vi "CmdExe.Run SystemExec and Wait, with Timeout.vi"() -> ()   [LabVIEW 2018]
uses:
  CmdConsole/CmdConsole.lvclass
  <vilib>/KATE/Time/Time Utils.lvlib
panel:
  out "Duration":dbl
  out "Std Out":string
  out "RtnCode":i32
  out "Std Error":string
  in  "Timeout(s)":dbl=1.0
  out "WaitForExit":bool
  out "HasExited":bool
  in  "Args":string
  out "error out":errorcluster
  in  "error in (no error)":errorcluster
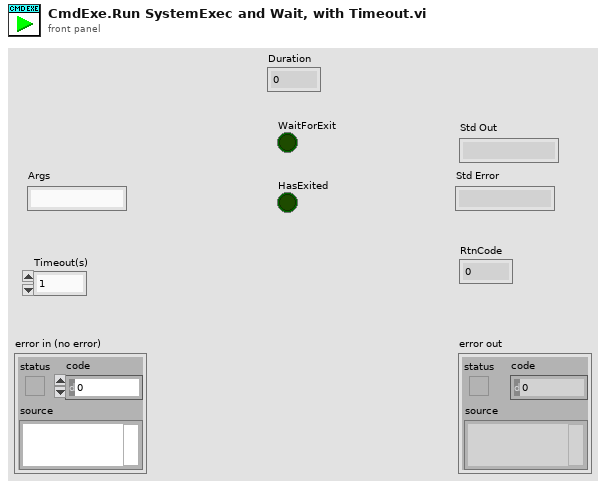
[diagram p1: front panel]
types:
  T1 = cluster{"StdOut":string, "StdErr":string, "RtnCode":i32}
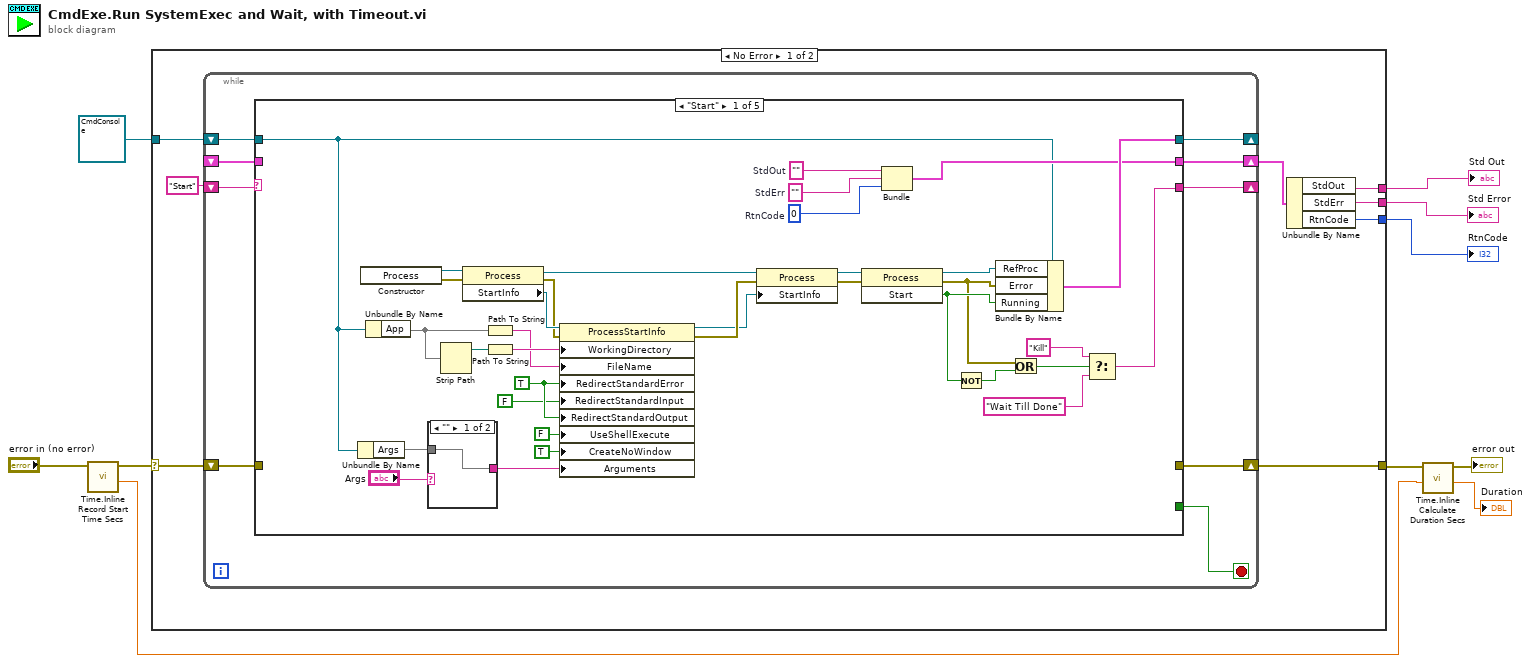
[diagram p0: block diagram]
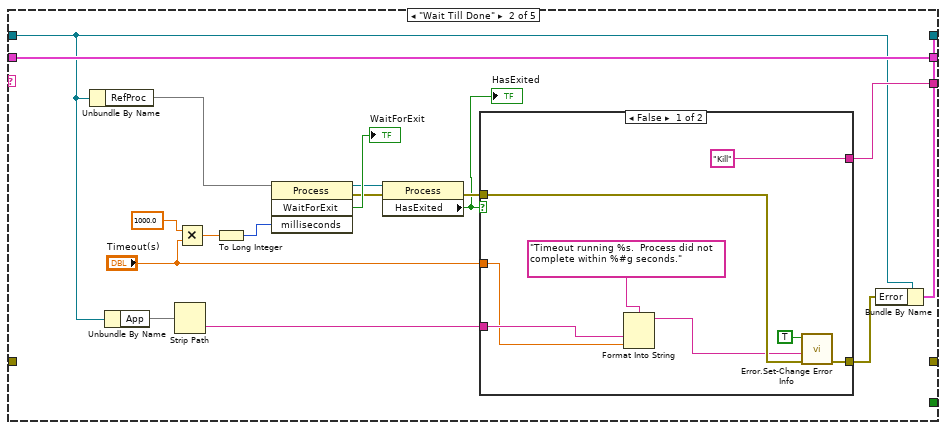
[diagram p3: hidden frame]
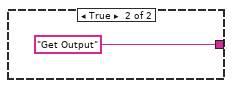
[diagram p4: hidden frame]
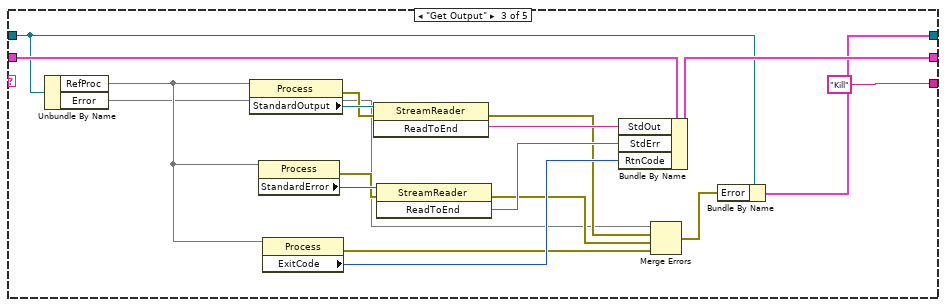
[diagram p5: hidden frame]
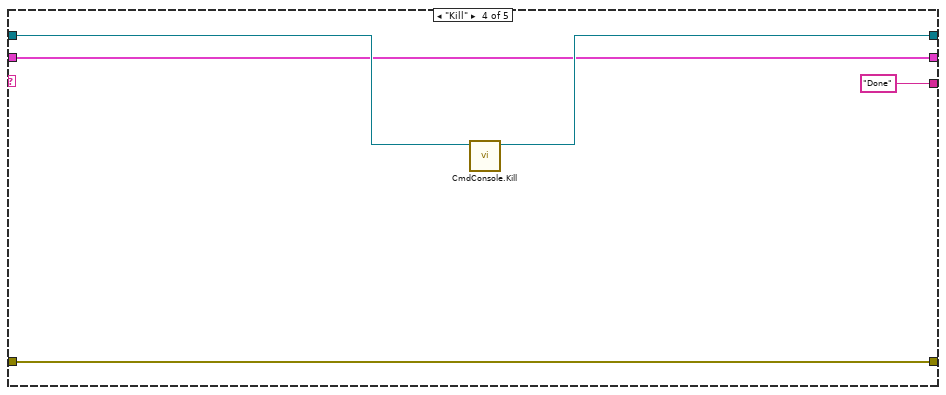
[diagram p6: hidden frame]
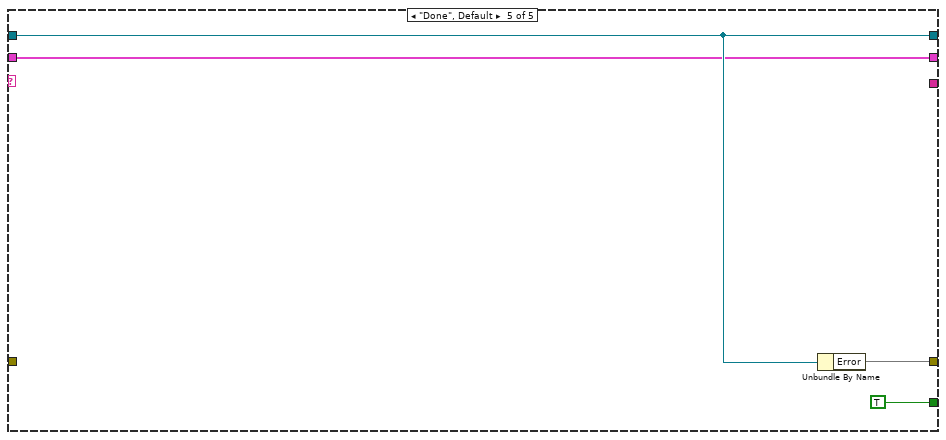
[diagram p7: hidden frame]
diagram:
  n1 = call <vilib>:"Time.Inline Record Start Time Secs.vi"("Error In Upper"="error in (no error)") -> ("Start(s)"=w2:dbl, "Error Out Upper"=w5:errorcluster)  [unwired: 8 in, 1 out]
  n2 = case shown="No Error" w5 {
    selector: w5 -> [w15 w118]
    tunnel: [w16 w118] -> w3
    tunnel: refnum<class "CmdConsole.lvclass"> refnum ("CmdConsole in") -> [w18 w117]
    tunnel: [w14 _] -> w9
    tunnel: [w12 _] -> w8
    tunnel: [w11 _] -> w7
    frame No Error {
      n3 = while {
        shift-right: [w26] -> _
        shift-left: w18 -> [w27]
        shift-right: [w24] -> _
        shift-left: "Start" -> [w25]
        shift-right: [w22] -> w16
        shift-left: w15 -> [w19]
        shift-right: [w21] -> w13
        shift-left: _ -> [w20]
        stop <- w23 stop-if-true
        n4 = case shown="\"Start\"" w25 {
          tunnel: w27 -> [w31 w65 w98 w112 w115]
          tunnel: [w45 w64 w97 w110 w115] -> w26
          tunnel: [w37 w76 "Kill" "Done" _] -> w24
          tunnel: [_ _ _ _ TRUE] -> w23
          tunnel: [_ _ _ w108 w114] -> w22
          tunnel: [w32 w71 w103 w109 w113] -> w21
          tunnel: w20 -> [_ w71 w104 w109 w113]
          tunnel: w19 -> [_ _ _ w108 _]
          frame "Start" {
            w33 = 0  # RtnCode
            w34 = ""  # StdErr
            w35 = ""  # StdOut
            w46 = TRUE ("UseShellExecute")
            n5 = Unbundle By Name(w31) -> ("Args"=w28)
            n6 = constructor class="Process"() -> (reference out=w61:refnum<k24>, error out=w60:errorcluster)  [unwired: 3 in, 1 out]
            n7 = Unbundle By Name(w31) -> ("App"=w47)
            n8 = case shown="\"\"" "Args" {
              selector: "Args" -> [_ w63]
              tunnel: [w62 w63] -> w29
              tunnel: w28 -> [w62 _]
              frame "" {
              }
              frame Default {
              }
            }
            n9 = Strip Path(path=w47) -> (stripped path=w50:path)  [unwired: 1 out]
            n10 = property class="Process"(reference=w61, error in=w60) -> (reference out=w53:refnum<k24>, error out=w54:errorcluster, "StartInfo"=w59:refnum<k24>)
            n11 = Path To String(path=w47) -> (string=w48:string)
            n12 = Path To String(path=w50) -> (string=w49:string)
            n13 = property class="ProcessStartInfo"(reference=w59, error in=w54, "WorkingDirectory"=w49, "FileName"=w48, "RedirectStandardError"=w46, "RedirectStandardInput"=FALSE ("UseShellExecute"), "RedirectStandardOutput"=w46, "UseShellExecute"=FALSE, "CreateNoWindow"=TRUE, "Arguments"=w29) -> (reference out=w55:refnum<k24>, error out=w56:errorcluster)
            n14 = property class="Process"(reference=w53, error in=w56, "StartInfo"=w55) -> (reference out=w52:refnum<k24>, error out=w51:errorcluster)
            n15 = invoke class="Process" method="Start"(reference=w52, error in=w51) -> (reference out=w44:refnum<k24>, error out=w41:errorcluster, "Start"=w43:bool)  [unwired: 1 in]
            n16 = Bundle("StdOut"=w35, "StdErr"=w34, "RtnCode"=w33) -> (w32:T1)  [unwired: 1 in]
            n17 = Not(x=w43) -> (.not. x?=w42:bool)
            n18 = Bundle By Name(cluster=w31, "RefProc"=w44, "Error"=w41, "Running"=w43) -> (w45:cluster{})
            n19 = Or(x=w41, y=w42) -> (x .or. y?=w40:bool)
            n20 = Select(t="Kill", s=w40, f="Wait Till Done") -> (s? t:f=w37:string)
          }
          frame "Wait Till Done" {
            n21 = Unbundle By Name(w65) -> ("RefProc"=w80)
            n22 = Unbundle By Name(w65) -> ("App"=w75)
            n23 = Strip Path(path=w75) -> (name=w74:string)  [unwired: 1 out]
            n24 = Multiply(x=1000.0 ("y"), y="Timeout(s)") -> (x*y=w79:dbl)
            n25 = To Long Integer(number=w79) -> (32bit integer=w78:i32)
            n26 = invoke class="Process" method="WaitForExit"(reference=w80, "milliseconds"=w78) -> (reference out=w70:refnum<k24>, error out=w68:errorcluster, "WaitForExit"=→"WaitForExit":bool)  [unwired: 2 in, 1 out]
            n27 = property class="Process"(reference=w70, error in=w68) -> (error out=w69:errorcluster, "HasExited"=w67:bool)  [unwired: 1 out]
            "HasExited" <- w67
            n28 = case shown="False" w67 {
              tunnel: ["Kill" "Get Output"] -> w76
              tunnel: w74 -> [w83 _]
              tunnel: w69 -> [w86 _]
              tunnel: [w85 _] -> w66
              tunnel: "Timeout(s)" -> [w82 _]
              frame False {
                n29 = Format Into String(format string="Timeout running %s.  Process did not complete within %#g seconds.", w83, w82) -> (resulting string=w81:string)  [unwired: 2 in, 1 out]
                n30 = call "Error.Set-Change Error Info.vi"("error in"=w86, "Description"=w81, "Set Error"=TRUE) -> ("error out"=w85:errorcluster)  [unwired: 8 in]
              }
              frame True {
              }
            }
            n31 = Bundle By Name(cluster=w65, "Error"=w66) -> (w64:cluster{})
          }
          frame "Get Output" {
            n32 = Unbundle By Name(w98) -> ("RefProc"=w100, "Error"=w90)
            n33 = property class="Process"(reference=w100) -> (error out=w96:errorcluster, "StandardOutput"=w106:refnum<k24>)  [unwired: 1 in, 1 out]
            n34 = property class="Process"(reference=w100) -> (error out=w95:errorcluster, "StandardError"=w102:refnum<k24>)  [unwired: 1 in, 1 out]
            n35 = property class="Process"(reference=w100) -> (error out=w94:errorcluster, "ExitCode"=w99:i32)  [unwired: 1 in, 1 out]
            n36 = invoke class="StreamReader" method="ReadToEnd"(reference=w106, error in=w96) -> (error out=w92:errorcluster, "ReadToEnd"=w105:string)  [unwired: 1 in, 1 out]
            n37 = invoke class="StreamReader" method="ReadToEnd"(reference=w102, error in=w95) -> (error out=w93:errorcluster, "ReadToEnd"=w101:string)  [unwired: 1 in, 1 out]
            n38 = Bundle By Name(cluster=w104, "StdOut"=w105, "StdErr"=w101, "RtnCode"=w99) -> (w103:T1)
            n39 = Merge Errors(w90, w92, w93, w94) -> (w91:errorcluster)
            n40 = Bundle By Name(cluster=w98, "Error"=w91) -> (w97:cluster{})
          }
          frame "Kill" {
            n41 = call "CmdConsole.Kill.vi"("CmdConsole in"=w112) -> ("CmdConsole out"=w110:refnum<class "CmdConsole.lvclass">)  [unwired: 9 in, 1 out]
          }
          frame "Done", Default {
            n42 = Unbundle By Name(w115) -> ("Error"=w114)
          }
        }
      }
      n43 = Unbundle By Name(w13) -> ("StdOut"=w14:string, "StdErr"=w12:string, "RtnCode"=w11:i32)
    }
    frame Error {
    }
  }
  "Std Error" <- w8
  "RtnCode" <- w7
  "Std Out" <- w9
  n44 = call <vilib>:"Time.Inline Calculate Duration Secs.vi"("Start(Sec)"=w2, "Error In Top"=w3) -> ("Duration(s)"=→"Duration":dbl, "Error Out Top"=→"error out":errorcluster)  [unwired: 7 in, 1 out]
